vi "DriveGetDist.vi"() -> (0 "Right dist":dbl, 1 "Left dist":dbl)   [LabVIEW 2020]
doc: "Gets left and right distance variables for drive"
uses:
  DriveGlobal.vi
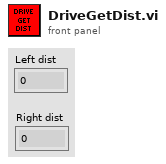
[diagram p1: front panel]
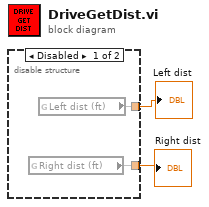
[diagram p0: block diagram]
diagram:
  n1 = disable-structure shown="Disabled" {
    disable-tunnel: [w4 _] -> w2
    disable-tunnel: [w3 _] -> w1
    frame Disabled {
      n2 = global read "DriveGlobal.vi" "Right dist (ft)"() -> (w3)
      n3 = global read "DriveGlobal.vi" "Left dist (ft)"() -> (w4)
    }
    frame Enabled {
    }
  }
  "Left dist" <- w2
  "Right dist" <- w1
